vi "GetRemote.vi"(6 "Legacy (f)?":bool, 8 "error in (no error)":errorcluster) -> (0 "error out":errorcluster, 2 "Remote":bool)   [LabVIEW 2011]
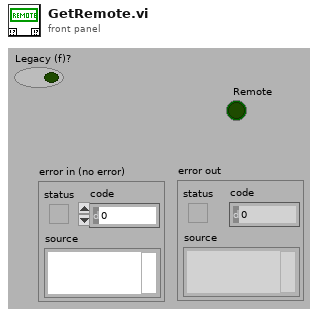
[diagram p1: front panel]
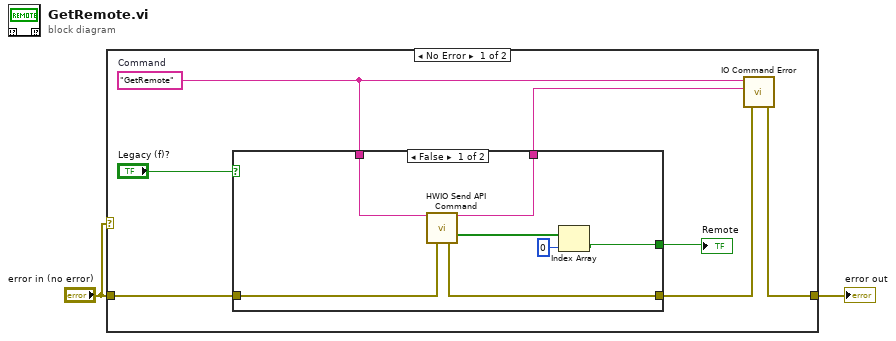
[diagram p0: block diagram]
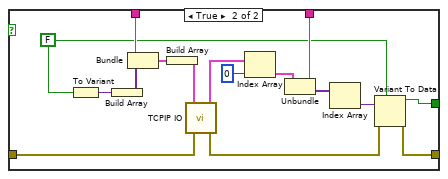
[diagram p2: hidden frame]
diagram:
  n1 = case shown="No Error" "error in (no error)" {
    tunnel: "error in (no error)" -> [w8 w33]
    tunnel: [w6 w33] -> w2
    frame No Error {
      w5 = "GetRemote"  # Command
      n2 = case shown="False" "Legacy (f)?" {
        tunnel: [w10 w28] -> w9
        tunnel: w8 -> [w16 w26]
        tunnel: [w15 w25] -> w7
        tunnel: w5 -> [w13 w24]
        tunnel: [w14 w23] -> w4
        frame False {
          n3 = call "HWIO Send API Command.vi"("Action"=w13, "error in (no error)"=w16) -> ("Action out"=w14:string, "Boolean out"=w12:bool[], "error out"=w15:errorcluster)  [unwired: 6 in, 5 out]
          n4 = Index Array(array=w12, index=0) -> (element=w10:bool)
        }
        frame True {
          w17 = FALSE
          n5 = To Variant(anything=w17) -> (Variant=w32:variant)
          n6 = Build Array(w32) -> (w31:variant[])
          n7 = Bundle("Command"=w24, w31) -> (w30:cluster{"Command":string, variant[]})  [unwired: 1 out]
          n8 = Build Array(w30) -> (w21:cluster{"Command":string, variant[]}[])
          n9 = call "TCPIP IO.vi"("error in (no error)"=w26, "Commands"=w21) -> ("error out"=w27:errorcluster, "Responses"=w22:cluster{string, variant[]}[])  [unwired: 1 in, 3 out]
          n10 = Index Array(array=w22, index=0) -> (element=w20:cluster{string, variant[]})
          n11 = Unbundle(w20) -> (w23:string, w19:variant[])
          n12 = Index Array(array=w19) -> (element=w18:variant)  [unwired: 1 in]
          n13 = Variant To Data(error in=w27, type=w17, Variant=w18) -> (data=w28:bool, error out=w25:errorcluster)
        }
      }
      "Remote" <- w9
      n14 = call "IO Command Error.vi"("error in (no error)"=w7, "Command Returned (\"\")"=w4, "Command Sent (\"\")"=w5) -> ("error out"=w6:errorcluster)  [unwired: 4 out]
    }
    frame Error {
    }
  }
  "error out" <- w2
